vi "LVClass_Camera set Parameter String.vi"(0 "Camera in":refnum<class "Camera.lvclass">, 7 "parameter_name":string, 9 "value":string, 11 "error in (no error)":errorcluster) -> (4 "Camera out":refnum<class "Camera.lvclass">, 15 "error out":errorcluster)   [LabVIEW 2020, in "Camera.lvclass"]
doc: "camera parameter setter for parameter of type E_TYPE_STRING.\n\n<B>cameraIn</B> : camera object.\n<B>cameraOut</B> : camera object.\n<B>parameter_name</B> : Name of the parameter.\n<B>value</B> : Value of the parameter."
uses:
  Camera.lvclass
  Camera.lvclass/Camera.ctl
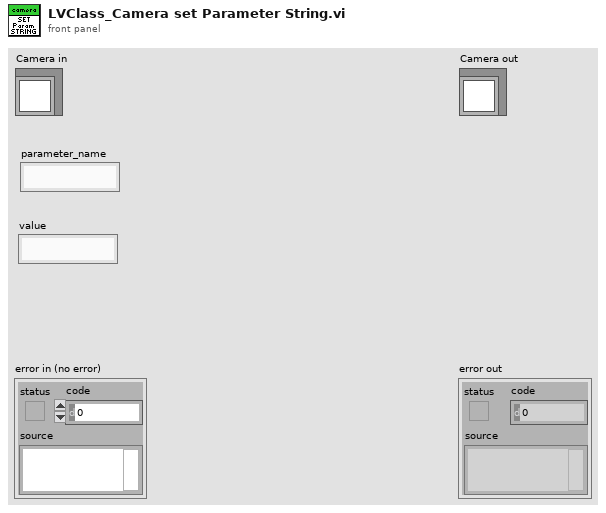
[diagram p1: front panel]
types:
  T1 = typedef "ClassID.ctl" = i64
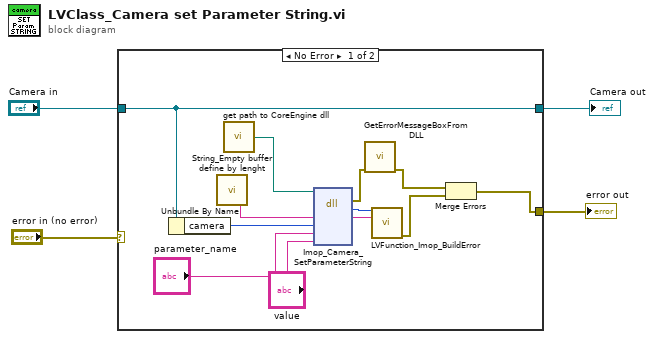
[diagram p0: block diagram]
diagram:
  n1 = case shown="No Error" "error in (no error)" {
    selector: "error in (no error)" -> [_ w18]
    tunnel: [w5 w18] -> w3
    tunnel: [w13 w17] -> w1
    tunnel: "Camera in" -> [w13 w17]
    frame No Error {
      n2 = Unbundle By Name(w13) -> ("camera"=w14:T1)
      n3 = call "String_Empty buffer define by lenght.vi"() -> ("Empty buffer"=w9:string)  [unwired: 1 in]
      n4 = call "get path to CoreEngine dll.vi"() -> ("path to wavekit library"=w12:path)  [unwired: 14 in, 1 out]
      n5 = dll-call lib="D:/2_trunk/Soft_haso/ImOpCoreEngine4_LV2011/DLLs/ImopEngine4_vc100.dll" fn="Imop_Camera_SetParameterString"(path in=w12, "message"=w9, "camera"=w14, "parameter_name"="parameter_name", "value"="value") -> (error out=w11:errorcluster, "return type"=w16:i32, "message"=w15:string)  [unwired: 5 in, 1 out]
      n6 = call "GetErrorMessageBoxFromDLL.vi"("error IN"=w11) -> ("error OUT"=w7:errorcluster)  [unwired: 10 in]
      n7 = call "LVFunction_Imop_BuildError.vi"("code"=w16, "String to Prepend to source (\"\")"=w15) -> ("error out"=w6:errorcluster)  [unwired: 13 in]
      n8 = Merge Errors(w7, w6) -> (w5:errorcluster)
    }
    frame Error {
    }
  }
  "error out" <- w3
  "Camera out" <- w1
